vi "Read EF Position.vi"(8 "error in (no error)":errorcluster, 11 "Simu Delta Robot in":refnum<class "Simu Delta Robot.lvclass">) -> (0 "error out":errorcluster, 2 "ef pos":dbl[](array[numeric]), 3 "Simu Delta Robot out":refnum<class "Simu Delta Robot.lvclass">)   [LabVIEW 2014, in "Simu Delta Robot.lvclass"]
uses:
  Simu Delta Robot.lvclass
  Simu Delta Robot.lvclass/Simu Delta Robot.ctl
  <vilib>/Analysis/7linalg.llb/Real Transpose Matrix.vi
  <vilib>/Analysis/baseanly.llb/A x Vector.vi
  <resource>/objmgr/LVODE.rc
  <vilib>/Analysis/NI_AALPro.lvlib
  <vilib>/Analysis/NI_AALBase.lvlib
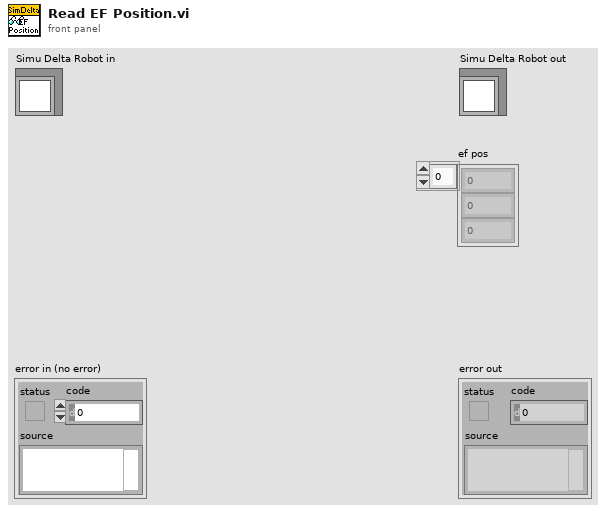
[diagram p1: front panel]
types:
  T1 = typedef "NI_Matrix.lvlib/RealMatrix.ctl" = dbl[][]
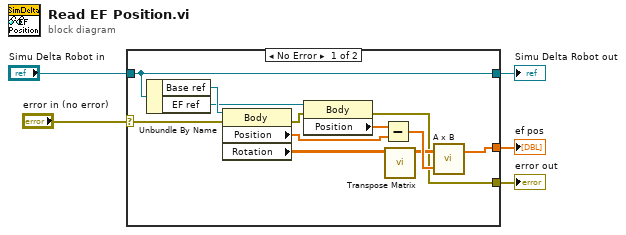
[diagram p0: block diagram]
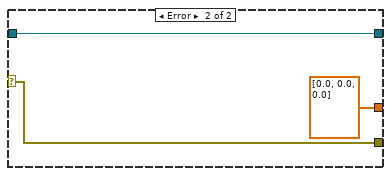
[diagram p2: hidden frame]
diagram:
  n1 = case shown="No Error" "error in (no error)" {
    selector: "error in (no error)" -> [w10 w19]
    tunnel: [w6 w19] -> w4
    tunnel: [w17 w20] -> w2
    tunnel: "Simu Delta Robot in" -> [w17 w20]
    tunnel: [w7 dbl[] [0.0, 0.0, 0.0] ("A x Vector")] -> w1
    frame No Error {
      n2 = Unbundle By Name(w17) -> ("Base ref"=w11:refnum<k20>, "EF ref"=w9:refnum<k20>)
      n3 = property class="Body"(reference=w11, error in=w10) -> (error out=w8:errorcluster, "Position"=w13:sgl[], "Rotation"=w14:sgl[][])  [unwired: 1 out]
      n4 = property class="Body"(reference=w9, error in=w8) -> (error out=w6:errorcluster, "Position"=w12:sgl[])  [unwired: 1 out]
      n5 = Subtract(x=w12, y=w13) -> (x-y=w16:sgl[])
      n6 = call-poly <vilib>:"Transpose Matrix.vi"("Input Matrix"=w14) -> ("Matrix Transpose"=w15:T1)  [unwired: 9 in, 1 out]
      n7 = call-poly <vilib>:"A x B.vi"("Vector"=w16, "A"=w15) -> ("A x Vector"=w7:dbl[])  [unwired: 1 out]
    }
    frame Error {
    }
  }
  "error out" <- w4
  "Simu Delta Robot out" <- w2
  "ef pos" <- w1
